vi "LCOS Init.vi"(0 "LCOS Display Queue":refnum<queue>, 2 "LCOS Displayed Image":T1, 3 "error in (no error)":errorcluster, 4 "LCOS Pattern Display.vi Name":string="LCOS Pattern Display_red.vi") -> (9 "error out":errorcluster)   [LabVIEW 2011]
uses:
  LCOS Pattern Display Actions.ctl
  <vilib>/vision/Image Controls.llb/IMAQ Image.ctl
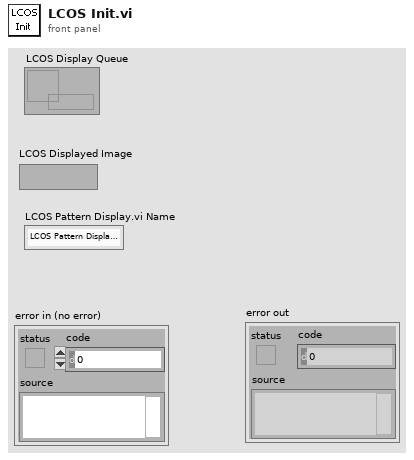
[diagram p1: front panel]
types:
  T1 = typedef "IMAQ Image.ctl" = refnum<image>
  T2 = typedef "LCOS Pattern Display Actions.ctl" = enum16{"Init", "Idle", "Update", "Exit"}
  T3 = cluster{"LCOS Pattern Display Actions":T2, "Data":variant}
  T4 = cluster{"LCOS Pattern Display Actions":T2, "Data":variant}[]
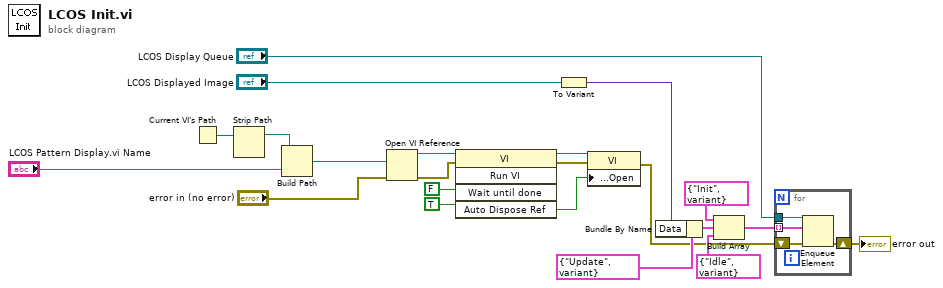
[diagram p0: block diagram]
diagram:
  w4 = TRUE ("Auto Dispose Reference")
  n1 = Current VI's Path() -> (path=w21:path)
  n2 = Strip Path(path=w21) -> (stripped path=w20:path)  [unwired: 1 out]
  n3 = Build Path(base path=w20, name or relative path="LCOS Pattern Display.vi Name") -> (appended path=w19:path)
  n4 = Open VI Reference(vi path=w19, error in (no error)="error in (no error)") -> (vi reference=w10:refnum<vi>, error out=w9:errorcluster)  [unwired: 4 in]
  n5 = invoke class="VI" method="Run VI"(reference=w10, error in=w9, "Wait until done"=FALSE ("Wait Until Done"), "Auto Dispose Ref"=w4) -> (reference out=w7:refnum<vi>, error out=w6:errorcluster)  [unwired: 1 in, 3 out]
  n6 = To Variant(anything="LCOS Displayed Image") -> (Variant=w15:variant)
  n7 = property class="VI"(reference=w7, error in=w6, "Front Panel.Open"=w4) -> (error out=w5:errorcluster)  [unwired: 1 out]
  n8 = Bundle By Name(cluster=T3 {"LCOS Pattern Display Actions"=enum."Update", "Data"=variant} ("element"), "Data"=w15) -> (w16:T3)
  n9 = Build Array(T3 {"LCOS Pattern Display Actions"=enum."Init", "Data"=variant} ("element"), w16, T3 {"LCOS Pattern Display Actions"=enum."Idle", "Data"=variant} ("element")) -> (w13:T4)
  n10 = for {
    tunnel: "LCOS Display Queue" -> [w24]
    tunnel: w13 -> [w23] mode=indexing
    shift-right: [w22] -> w14
    shift-left: w5 -> [w25]
    n11 = Enqueue Element(queue=w24, element=w23, error in (no error)=w25) -> (error out=w22:errorcluster)  [unwired: 1 in, 2 out]
  }
  "error out" <- w14
